vi "Set Reset Allarmi.vi"(7 "Lista allarmi":string[](array[string]), 10 "Reset":bool, 11 "Array allarmi":bool[](array[boolean])) -> (1 "Lista allarmi":string[](array[string]), 2 "Allarme?":bool, 3 "Allarmi out":bool[](array[boolean]))   [LabVIEW 2019]
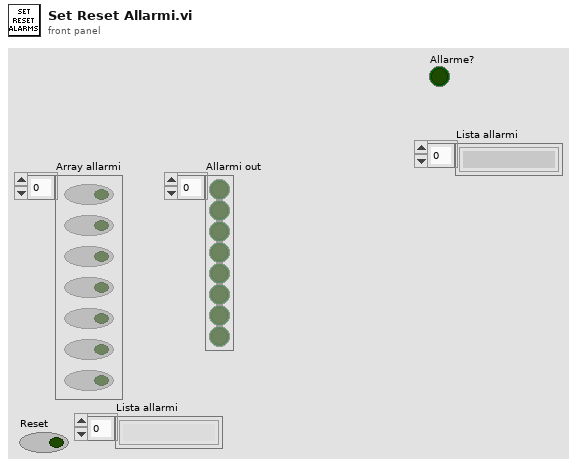
[diagram p1: front panel]
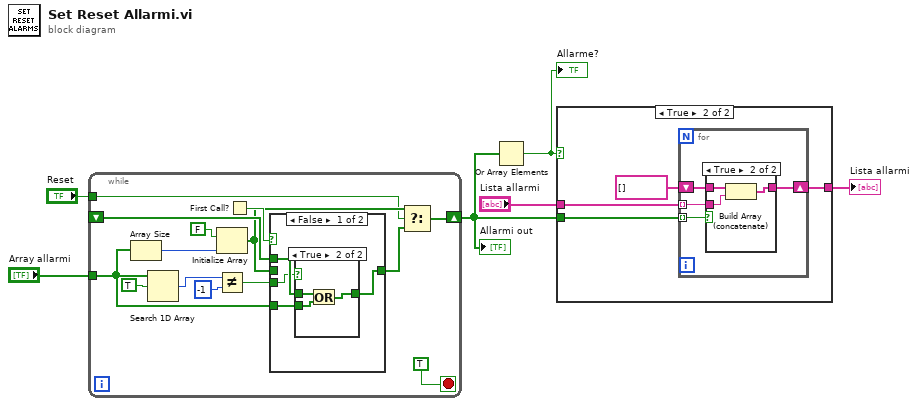
[diagram p0: block diagram]
diagram:
  n1 = while {
    shift-right: [w18] -> w1
    shift-left: _ -> [w17]
    tunnel: "Array allarmi" -> [w11]
    tunnel: "Reset" -> [w12]
    stop <- TRUE stop-if-true
    n2 = Array Size(array=w11) -> (size(s)=w15:i32)
    n3 = Search 1D Array(1D array=w11, element=TRUE) -> (index of element=w9:i32)  [unwired: 1 in]
    n4 = Initialize Array(FALSE ("x != 0?"), w15) -> (w13:bool[])
    n5 = Not Equal?(x=w9, y=-1) -> (x != y?=w7:bool)
    n6 = First Call?() -> (First Call?: T/F=w14:bool)
    n7 = case shown="False" w14 {
      tunnel: [w24 w29] -> w19
      tunnel: w17 -> [w23 _]
      tunnel: w7 -> [w22 _]
      tunnel: w11 -> [w21 _]
      tunnel: w13 -> [_ w29]
      frame False {
        n8 = case shown="True" w22 {
          tunnel: [w25 w26] -> w24
          tunnel: w21 -> [_ w28]
          tunnel: w23 -> [w25 w27]
          frame False {
          }
          frame True {
            n9 = Or(x=w27, y=w28) -> (x .or. y?=w26:bool[])
          }
        }
      }
      frame True {
      }
    }
    n10 = Select(t=w13, s=w12, f=w19) -> (s? t:f=w18:bool[])
  }
  "Allarmi out" <- w1
  n11 = Or Array Elements(Boolean array=w1) -> (logical OR=w4:bool)
  "Allarme?" <- w4
  n12 = case shown="True" w4 {
    tunnel: "Lista allarmi" -> [_ w33]
    tunnel: w1 -> [_ w32]
    tunnel: [_ w30] -> w3
    frame False {
    }
    frame True {
      n13 = for {
        tunnel: w33 -> [w35] mode=indexing
        tunnel: w32 -> [w37] mode=indexing
        shift-right: [w34] -> w30
        shift-left: string[] [] -> [w36]
        n14 = case shown="True" w37 {
          tunnel: w36 -> [w38 w41]
          tunnel: w35 -> [_ w40]
          tunnel: [w38 w39] -> w34
          frame False {
          }
          frame True {
            n15 = Build Array (concatenate)(w41, w40) -> (w39:string[])
          }
        }
      }
    }
  }
  "Lista allarmi" <- w3
